vi "dfd_FXP Lattice AR (normalized) with IS.vi"(6 "state in":i64[](array[numeric]), 7 "FXPOPs":T5[](array[typedef]) {"source" items=["Coef a/k"=0, "Coef b/v"=7, "Input"=1, "Output"=2, "Multiplicand"=3, "Product"=4, "Sum"=5, "Delay"=6, "Gain"=8]}, 8 "filtering statistics in":T4(array[cluster]) {"statistics information"."min value" format="%.2f"; "statistics information"."max value" format="%.2f"; "Quantizer Source" items=["Coefficients a/k"=0, "Coefficients b/v"=7, "Input"=1, "Output"=2, "Multiplicand"=3, "Product"=4, "Sum"=5, "Delay"=6]}, 10 "coef k & ^k":T7, 11 "X":T7) -> (0 "filtering statistics out":T4(array[cluster]) {"statistics information"."min value" format="%.2f"; "statistics information"."max value" format="%.2f"; "Quantizer Source" items=["Coefficients a/k"=0, "Coefficients b/v"=7, "Input"=1, "Output"=2, "Multiplicand"=3, "Product"=4, "Sum"=5, "Delay"=6]}, 3 "filtered X":T7, 4 "state out":i64[](array[numeric]))   [LabVIEW 2017, in "NI_DigFilter_FXP.lvlib"]
uses:
  <vilib>/addons/Digital Filter Design/NI_DigFilter_FXP.lvlib
  <vilib>/addons/Digital Filter Design/_Objects.llb/dfd_DFXP Data Type (vector).ctl
  <vilib>/addons/Digital Filter Design/_Objects.llb/dfd_DFXP Operation Parameter.ctl
  <vilib>/addons/Digital Filter Design/_Objects.llb/dfd_Internal Quantization Srcs.ctl
  <vilib>/addons/Digital Filter Design/_Objects.llb/DFD Quantization Sources.ctl
  <vilib>/addons/Digital Filter Design/_Objects.llb/DFD FXP Statistics Data.ctl
  <vilib>/addons/Digital Filter Design/_Objects.llb/dfd_DFXP Data Type (scaler).ctl
  <vilib>/addons/Digital Filter Design/NI_DigFilterLicensed.lvlib
panel:
  in  "DFXP Value":T1={"value"=0, "wl"=0, "iwl"=0, "Signed"=TRUE} {"value" format="%.0x"}
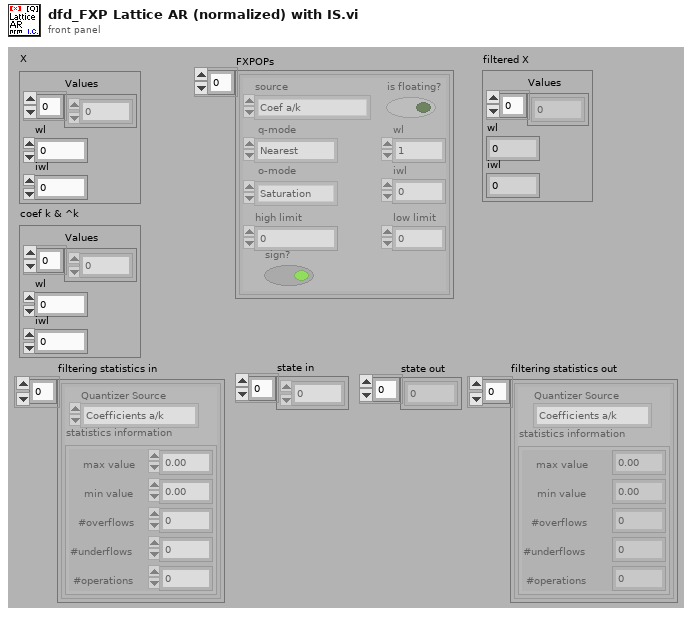
[diagram p1: front panel]
types:
  T1 = typedef "dfd_DFXP Data Type (scaler).ctl" = cluster{"value":i64, "wl":i16, "iwl":i16, "Signed":bool}
  T2 = typedef "NI_DigFilterLicensed.lvlib/DFD Quantization Sources.ctl" = u16
  T3 = typedef "NI_DigFilterLicensed.lvlib/DFD FXP Statistics Data.ctl" = cluster{"max value":ext, "min value":ext, "#overflows":i32, "#underflows":i32, "#operations":i32}
  T4 = cluster{"Quantizer Source":T2, "statistics information":T3}[]
  T5 = typedef "dfd_DFXP Operation Parameter.ctl" = cluster{"source":T6, "is floating?":bool, "o-mode":enum16{"Saturation", "Wrap"}, "q-mode":enum16{"Nearest", "Truncation"}, "wl":i16, "high limit":i64, "low limit":i64, "iwl":i16, "sign?":bool}
  T6 = typedef "NI_DigFilterLicensed.lvlib/dfd_Internal Quantization Srcs.ctl" = u16
  T7 = typedef "dfd_DFXP Data Type (vector).ctl" = cluster{"Values":i64[], "wl":i16, "iwl":i16}
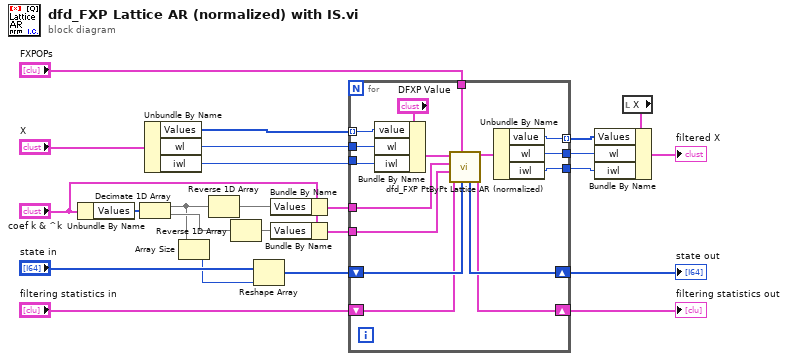
[diagram p0: block diagram]
diagram:
  n1 = Unbundle By Name("coef k & ^k") -> ("Values"=w11:i64[])
  n2 = Decimate 1D Array(w11) -> (w18:i64[], w21:i64[])
  n3 = Unbundle By Name("X") -> ("Values"=w7:i64[], "wl"=w6:i16, "iwl"=w5:i16)
  n4 = Array Size(array=w18) -> (size(s)=w15:i32)
  n5 = Reverse 1D Array(array=w18) -> (reversed array=w19:i64[])
  n6 = Reverse 1D Array(array=w21) -> (reversed array=w20:i64[])
  n7 = Reshape Array("state in", w15) -> (w23:i64[])
  n8 = Bundle By Name(cluster="coef k & ^k", "Values"=w19) -> (w10:T7)
  n9 = Bundle By Name(cluster="coef k & ^k", "Values"=w20) -> (w9:T7)
  n10 = for {
    tunnel: w7 -> [w40] mode=indexing
    tunnel: w10 -> [w37]
    shift-right: [w35] -> w14
    shift-left: w23 -> [w36]
    tunnel: w9 -> [w34]
    tunnel: [w27] -> w17 mode=indexing
    tunnel: "FXPOPs" -> [w38]
    shift-right: [w32] -> w12
    shift-left: "filtering statistics in" -> [w33]
    tunnel: w6 -> [w29]
    tunnel: w5 -> [w28]
    tunnel: [w26] -> w2
    tunnel: [w25] -> w1
    n11 = Bundle By Name(cluster="DFXP Value", "value"=w40, "wl"=w29, "iwl"=w28) -> (w31:T1)
    n12 = call <vilib>:"dfd_FXP PtByPt Lattice AR (normalized).vi"("state in"=w36, "FXPOPs"=w38, "filtering statistics in"=w33, "coef ^k[M..1]"=w34, "coef k[M..1]"=w37, "x"=w31) -> ("filtering statistics out"=w32:T4, "filtered x"=w39:T1, "state out"=w35:i64[])  [unwired: 3 out]
    n13 = Unbundle By Name(w39) -> ("value"=w27:i64, "wl"=w26:i16, "iwl"=w25:i16)
  }
  "state out" <- w14
  "filtering statistics out" <- w12
  n14 = local read "X"() -> (w3:T7)
  n15 = Bundle By Name(cluster=w3, "Values"=w17, "wl"=w2, "iwl"=w1) -> (→"filtered X":T7)
